vi "Set URL.vi"(0 "GMaps API in":refnum<class "GMaps API.lvclass">, 1 "URL":T1={"Street"="", "State"="", "City"=" ", "X"=0, "Y"=0, "Map Format"="hybrid", "Zoom"=0}, 5 "error in (no error)":errorcluster) -> (14 "GMaps API out":refnum<class "GMaps API.lvclass">, 19 "error out":errorcluster)   [LabVIEW 2016, in "GMaps API.lvclass"]
doc: "Sets Google Static Maps API URLs and the available parameters."
uses:
  GMaps API.lvclass
  Controls/URL.ctl
  GMaps API.lvclass/GMaps API.ctl
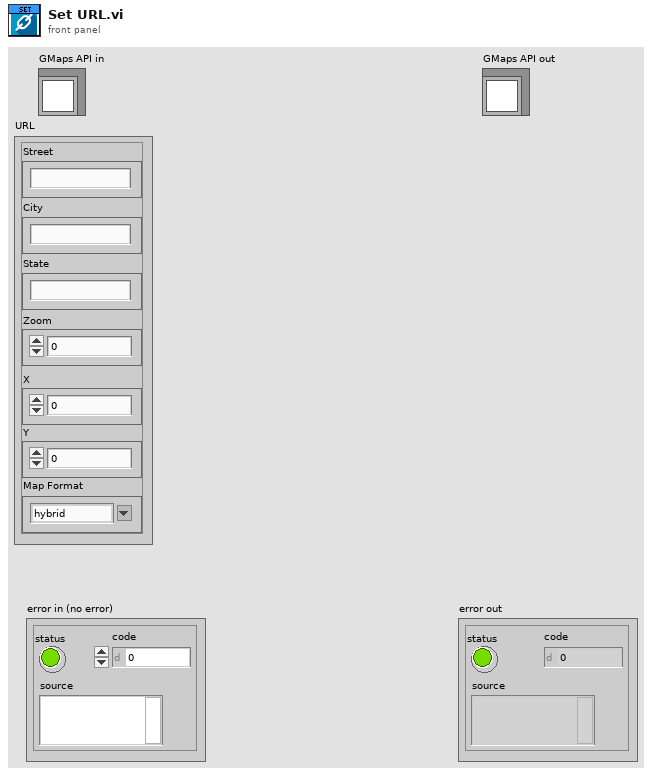
[diagram p1: front panel]
types:
  T1 = typedef "GMaps API.lvclass/URL.ctl" = cluster{"Street":string, "State":string, "City":string, "X":u32, "Y":u32, "Map Format":string, "Zoom":u64}
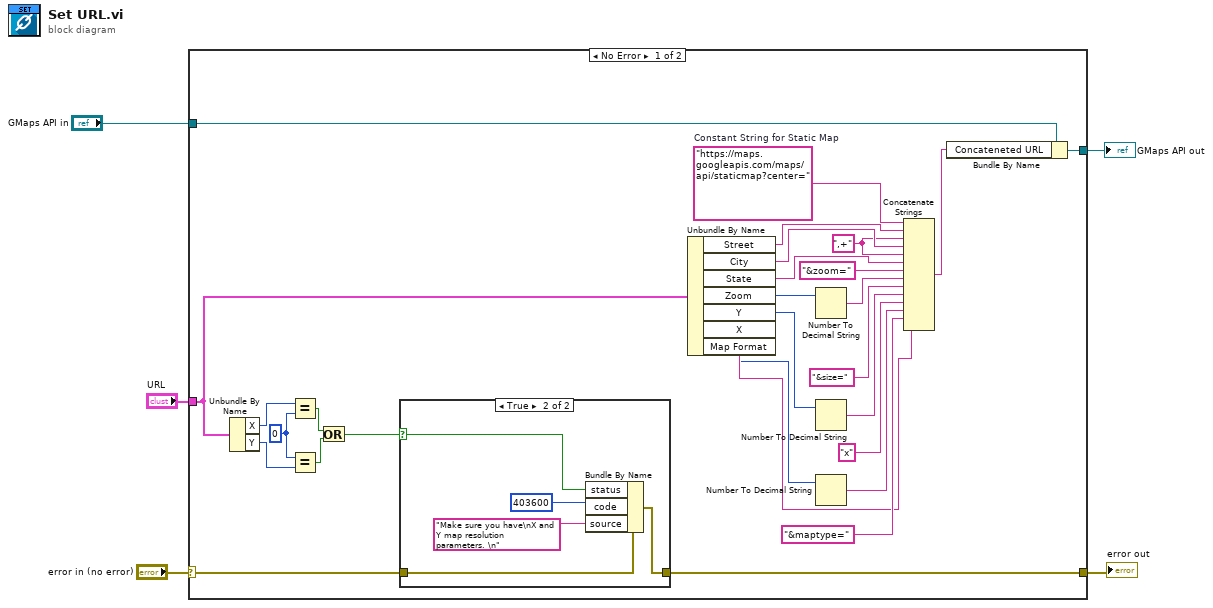
[diagram p0: block diagram]
diagram:
  n1 = case shown="No Error" "error in (no error)" {
    selector: "error in (no error)" -> [w8 w41]
    tunnel: [w7 w41] -> w4
    tunnel: [w32 w40] -> w2
    tunnel: "GMaps API in" -> [w33 w40]
    tunnel: "URL" -> [w6 _]
    frame No Error {
      w10 = u32 0
      w21 = ",+" ("string")
      w27 = "https://maps.googleapis.com/maps/api/staticmap?center="  # Constant String for Static Map
      n2 = Unbundle By Name(w6) -> ("X"=w11:u32, "Y"=w12:u32)
      n3 = Equal?(x=w11, y=w10) -> (x = y?=w14:bool)
      n4 = Equal?(x=w10, y=w12) -> (x = y?=w13:bool)
      n5 = Or(x=w14, y=w13) -> (x .or. y?=w9:bool)
      n6 = case shown="True" w9 {
        selector: w9 -> [_ w37]
        tunnel: w8 -> [w34 w38]
        tunnel: [w34 w39] -> w7
        frame False {
        }
        frame True {
          n7 = Bundle By Name(cluster=w38, "status"=w37, "code"=403600 ("error code (0)"), "source"="Make sure you have\nX and Y map resolution parameters. \n" ("error message (\"\")")) -> (w39:errorcluster)
        }
      }
      n8 = Unbundle By Name(w6) -> ("Street"=w25:string, "City"=w24:string, "State"=w23:string, "Zoom"=w19:u64, "Y"=w18:u32, "X"=w16:u32, "Map Format"=w22:string)
      n9 = Number To Decimal String(number=w19) -> (decimal integer string=w20:string)  [unwired: 1 in]
      n10 = Number To Decimal String(number=w18) -> (decimal integer string=w17:string)  [unwired: 1 in]
      n11 = Number To Decimal String(number=w16) -> (decimal integer string=w15:string)  [unwired: 1 in]
      n12 = Concatenate Strings(w27, w25, w21, w24, w21, w23, "&zoom=", w20, "&size=", w17, "x", w15, "&maptype=" ("string"), w22) -> (w26:string)
      n13 = Bundle By Name(cluster=w33, "Concateneted URL"=w26) -> (w32:refnum<class "GMaps API.lvclass">)
    }
    frame Error {
    }
  }
  "error out" <- w4
  "GMaps API out" <- w2
